vi "Insert End Lines.vi"(8 "error in (no error)":errorcluster, 10 "max chars in line":i32, 11 "string in":string) -> (0 "error out":errorcluster, 3 "string with end lines":string)   [LabVIEW 2017]
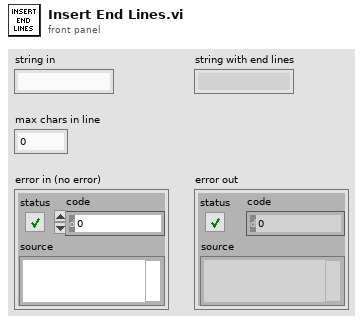
[diagram p1: front panel]
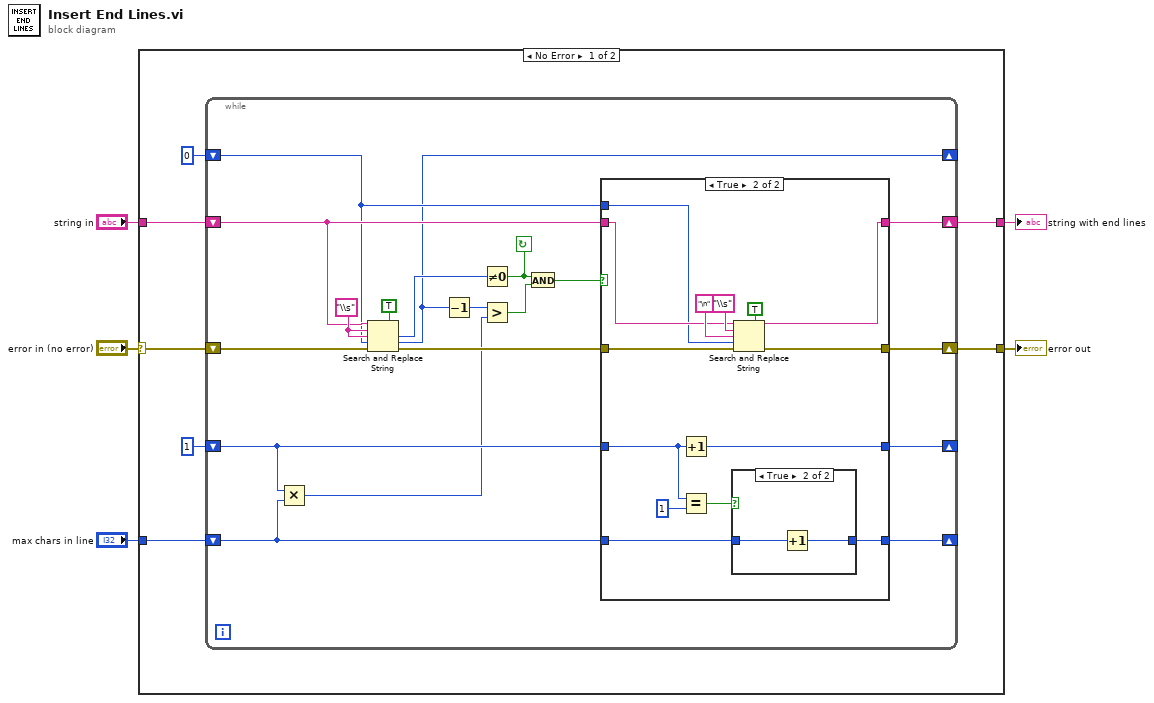
[diagram p0: block diagram]
diagram:
  n1 = case shown="No Error" "error in (no error)" {
    selector: "error in (no error)" -> [w8 w54]
    tunnel: "string in" -> [w12 w53]
    tunnel: [w10 w53] -> w4
    tunnel: [w7 w54] -> w2
    tunnel: "max chars in line" -> [w6 _]
    frame No Error {
      n2 = while {
        shift-right: [w15] -> _
        shift-left: 0 -> [w21]
        shift-right: [w25] -> w10
        shift-left: w12 -> [w24]
        shift-right: [w23] -> _
        shift-left: 1 -> [w22]
        shift-right: [w16] -> _
        shift-left: w6 -> [w17]
        shift-right: [w14] -> w7
        shift-left: w8 -> [w13]
        stop <- w26 continue-if-true
        w31 = "\\s" ("search string")
        n3 = Multiply(x=w22, y=w17) -> (x*y=w18:i32)
        n4 = Search and Replace String(multiline?=TRUE ("multiline? (F)"), input string=w24, search string=w31, replace string=w31, offset=w21, error in=w13) -> (number of replacements=w29:i32, offset past replacement=w15:i32, error out=w27:errorcluster)  [unwired: 2 in, 1 out]
        n5 = Decrement(x=w15) -> (x-1=w20:i32)
        n6 = Not Equal To 0?(x=w29) -> (x != 0?=w26:bool)
        n7 = Greater?(x=w20, y=w18) -> (0:w19:bool)
        n8 = And(x=w26, y=w19) -> (x .and. y?=w28:bool)
        n9 = case shown="True" w28 {
          tunnel: w24 -> [w35 w47]
          tunnel: w27 -> [w32 w46]
          tunnel: [w35 w44] -> w25
          tunnel: [w34 w43] -> w23
          tunnel: w22 -> [w34 w41]
          tunnel: w21 -> [_ w42]
          tunnel: w17 -> [w33 w38]
          tunnel: [w33 w37] -> w16
          tunnel: [w32 w36] -> w14
          frame False {
          }
          frame True {
            n10 = Increment(x=w41) -> (x+1=w43:i32)
            n11 = Equal?(x=w41, y=1) -> (x = y?=w39:bool)
            n12 = case shown="True" w39 {
              tunnel: w38 -> [w50 w52]
              tunnel: [w50 w51] -> w37
              frame False {
              }
              frame True {
                n13 = Increment(x=w52) -> (x+1=w51:i32)
              }
            }
            n14 = Search and Replace String(multiline?=TRUE ("multiline? (F)"), input string=w47, search string="\\s", replace string="\n" ("replace string (\"\")"), offset=w42, error in=w46) -> (result string=w44:string, error out=w36:errorcluster)  [unwired: 2 in, 2 out]
          }
        }
      }
    }
    frame Error {
    }
  }
  "string with end lines" <- w4
  "error out" <- w2
